vi "Validate Checksum.vi"(11 "bytes in":string) -> (2 "Boolean":bool, 3 "bytes out":string)   [LabVIEW 2019, in "PGC2D.lvlib"]
uses:
  PGC2D.lvlib
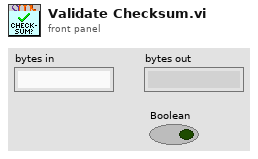
[diagram p1: front panel]
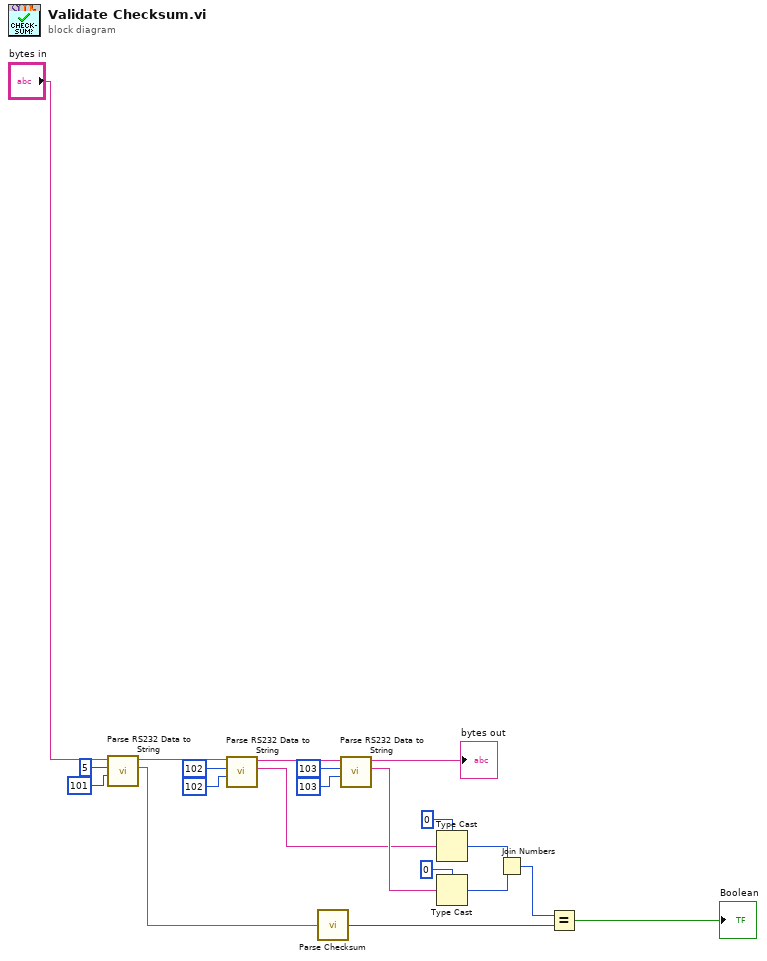
[diagram p0: block diagram]
diagram:
  n1 = call "Parse RS232 Data to String.vi"("AML end byte"=101, "AML start byte"=5, "bytes in"="bytes in") -> ("string data"=w14:string, "bytes out"=w4:string)  [unwired: 7 in]
  n2 = call "Parse RS232 Data to String.vi"("AML end byte"=102, "AML start byte"=102, "bytes in"=w4) -> ("string data"=w13:string, "bytes out"=w6:string)  [unwired: 7 in]
  n3 = call "Parse Checksum.vi"("bytes 5 - 101"=w14) -> ("checksum"=w16:u16)
  n4 = call "Parse RS232 Data to String.vi"("AML end byte"=103, "AML start byte"=103, "bytes in"=w6) -> ("string data"=w17:string, "bytes out"=→"bytes out":string)  [unwired: 7 in]
  n5 = Type Cast(type=u8 0 ("checksum"), x=w13) -> (*(type *) &x=w18:u8)
  n6 = Type Cast(type=u8 0 ("checksum"), x=w17) -> (*(type *) &x=w19:u8)
  n7 = Join Numbers(hi=w18, lo=w19) -> ((hi.lo)=w15:u16)
  n8 = Equal?(x=w15, y=w16) -> (x = y?=→"Boolean":bool)
